vi "Get kind of part.vi"(9 "Element":string, 11 "File Path":path) -> (1 "Element definiton out":string)   [LabVIEW 2021, in "Stack.lvclass"]
uses:
  Stack.lvclass
  <vilib>/Utility/file.llb/Read Delimited Spreadsheet (string).vi
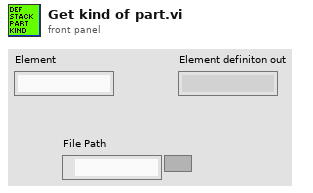
[diagram p1: front panel]
types:
  T1 = typedef "File Paths.ctl" = cluster{"Glue Pattern Folder":path, "Carrier Tray Folder":path, "Pick Up Tool Fixture Folder":path, "Components Folder":path, "Bellows Tool Offset.txt":path, "Pick Up Tool Offset.txt":path, "Dispense Tip Offset.txt":path, "Log Files":path, "Gantry Assembly Map.txt":path, "Syringe and offset map.txt":path, "Controllers Folder":path, "Local dbase config":path}
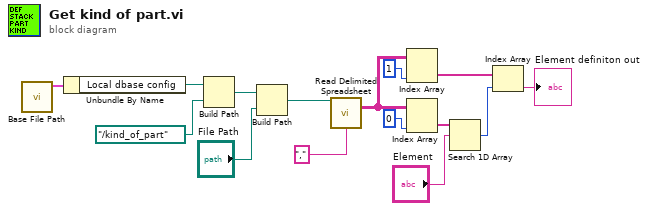
[diagram p0: block diagram]
diagram:
  n1 = call "Base File Path.vi"() -> ("Paths Out"=w15:T1)  [unwired: 11 in]
  n2 = Unbundle By Name(w15) -> ("Local dbase config"=w14:path)
  n3 = Build Path(base path=w14, name or relative path=path "../kind_of_part") -> (appended path=w12:path)
  n4 = Build Path(base path=w12, name or relative path="File Path") -> (appended path=w10:path)
  n5 = call-poly <vilib>:"Read Delimited Spreadsheet.vi"("file path (dialog if empty)"=w10, "delimiter (\\t)"="," ("delimiter (\\t)")) -> ("all rows"=w8:string[][])  [unwired: 8 in, 5 out]
  n6 = Index Array(array=w8, index (col)=1 ("disabled index (col)")) -> (element=w3:string[])  [unwired: 1 in]
  n7 = Index Array(array=w8, index (col)=0 ("disabled index (col)")) -> (element=w5:string[])  [unwired: 1 in]
  n8 = Search 1D Array(1D array=w5, element="Element") -> (index of element=w2:i32)  [unwired: 1 in]
  n9 = Index Array(array=w3, index=w2) -> (element=→"Element definiton out":string)
